vi "Obj To DVR.vi"(3 "signal configuration":refnum<class "SV Sinusoid.lvclass">) -> (0 "error_out":errorcluster, 1 "dataValueReference":u32)   [LabVIEW 2021]
uses:
  <vilib>/addons/_NISVFA/_Generation/Signal Generation/SV Sinusoid/SV Sinusoid.lvclass
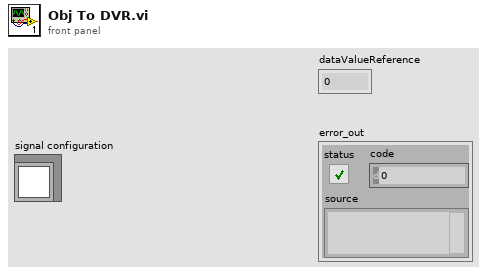
[diagram p1: front panel]
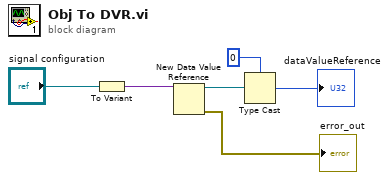
[diagram p0: block diagram]
diagram:
  n1 = To Variant(anything="signal configuration") -> (Variant=w6:variant)
  n2 = New Data Value Reference(data value=w6) -> (data value reference=w5:refnum<data-value>, error out=→"error_out":errorcluster)  [unwired: 1 in]
  n3 = Type Cast(type=u32 0 ("n"), x=w5) -> (*(type *) &x=→"dataValueReference":u32)
